vi "Funcion_LEER.vi"() -> ()   [LabVIEW 2016]
uses:
  microchip_solutions_v2013-06-15/USB/Tools/MCHPUSB Custom Driver/Mpusbapi/Dll/Borland_C/mpusbapi.dll
panel:
  out "subarray":bool[](array[boolean])
  out "plength*":i32
  out "pData*":i32
  in  "PIPE IN":i32
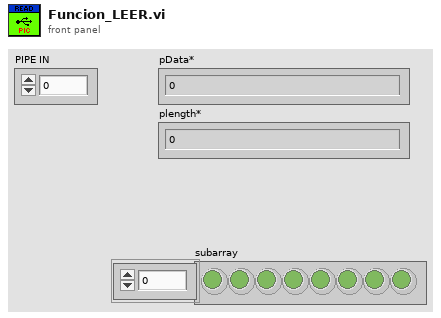
[diagram p1: front panel]
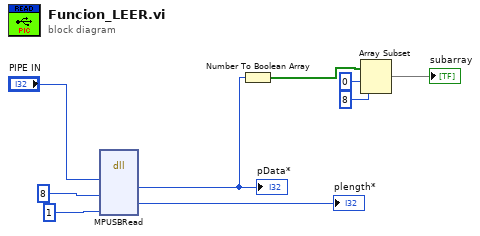
[diagram p0: block diagram]
diagram:
  n1 = dll-call lib="C:/microchip_solutions_v2013-06-15/USB/Tools/MCHPUSB Custom Driver/Mpusbapi/Dll/Borland_C/mpusbapi.dll" fn="MPUSBRead"("PIPE IN"="PIPE IN", "dwlen"=8, "dwMilliseconds"=1) -> ("pData*"=w2:i32, "plength"=→"plength*":i32)  [unwired: 9 in, 2 out]
  "pData*" <- w2
  n2 = Number To Boolean Array(number=w2) -> (Boolean array=w3:bool[])
  n3 = Array Subset(array=w3, index=0, length=8) -> (→"subarray":bool[])
